vi "Player Info.vi"(11 "Experience in":refnum<class "Experience.lvclass">) -> (0 "Defeat Speech":string, 1 "Victory Speech":string, 2 "Name":string, 3 "Experience out":refnum<class "Experience.lvclass">)   [LabVIEW 2015, in "Experience.lvclass"]
uses:
  Experience.lvclass
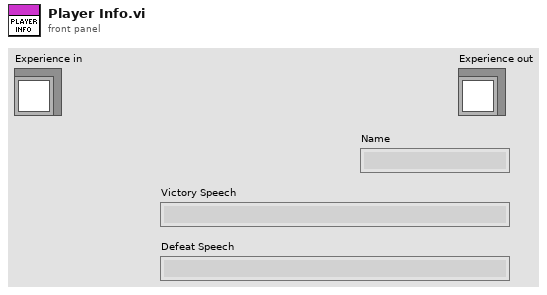
[diagram p1: front panel]
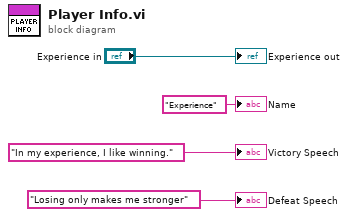
[diagram p0: block diagram]
diagram:
  "Experience out" <- "Experience in"
  "Name" <- "Experience" ("Name")
  "Victory Speech" <- "In my experience, I like winning." ("Victory Speech")
  "Defeat Speech" <- "Losing only makes me stronger" ("Victory Speech")
